vi "Main_16b_DNAtts for speed compare.vi"() -> ()   [LabVIEW 2023]
uses:
  ENUM_Direction.ctl
  07240289-bc54-4016-8294-605637801abb.vi
panel:
  out "x-y":i32
  out "answer":i32
  in  "Puzzle":string="\\.......................|..-.............../../.......|...............\\.\\.....|..../.............|............\n........................../....../..............................-............-.-..--.........-...........\\/...\n....\\............../...........-...-......|.............................\\...............-........-....|.......\n......\\....|................./.\\................/..................../.......................|..\\......-......\n.................../..................-./.................../.....-...................|......\\.......|\\...\\./.\n.....|........../....................\\../..\\.../.\\.......-.............\\...........\\......|.\\..-..........-...\n..../............/.....\\...................../..--\\........|......\\....-...|.-...../......-........../........\n..............\\.-............./........./....|\\.......\\..........|.................|.|.................-......\n.....|..........-................-.../..........-........................\\.......|.........................-..\n.|.-......./....................\\........-.............../..\\.|.-\\...........\\./.................-............\n................|/............................../..-.\\..................-..../../...../.../..../..........|...\n........................./.....................\\..\\....-....../-.....................\\|.........././.-........\n...\\.....................-...../|............--......-..|...../.....|......|.../.\\....|.............\\|.......\\\n.........-...-.....|.........../...-/........|......./|............-.......-.....\\.............\\|....../......\n.....|...|.................|...../.............|.................../..........\\|..\\......|..|....-............\n...........................-.........\\......\\.............\\...................-.....-.\\.......-.....|.........\n.................-.............-......./.............-..\\./......|....-..-..........-....-............\\.......\n.\\..\\.......-......|........................\\.............-.......................|.........|\\.|..\\......--/..\n..........-.....||--........|........-....../...........|../...-.........../.....-.\\..........|.......-.......\n..........\\..........|..................\\.................-..../............/..........|.......-........../...\n..--......../..........-..|........./.........-...../........-.................|..\\............../.....-......\n.....\\.............|...../......../............./||..........................\\............|...................\n..-.................-|..-....................\\.................|...\\.....\\............./......-.......\\.......\n............-../......\\...../.-....-.....-....-./../......\\..|..|............................|.../..|.........\n-................./................................................|...............|....|.....-.....|....../..\n...........-...................|...........\\.......-..\\.......-...........|..-....../........|...............|\n.........|...|-........../...-..........|.........\\.....||......./....|...............\\......-......\\...../...\n....|.........|............\\.-.......................................-.......................|.-..|.\\...\\.-...\n.|....|....-/....................\\\\..........................|........\\|...|..............\\..|......-.\\../....\n..|.\\......|..../.....|.......-....................|.\\..\\............/......................|.....\\../../.....\n.......|\\\\.\\/......................./.............|................../.........|.....\\-.......................\n......................................../.../................\\-..............-................./......\\.......\n............../............/\\......./........................./......|............\\/..........................\n......./................|......../.........-............\\.../.|....../....|...../..../......../...............\n...................|............-\\........../...\\.......\\....\\.....-.........-./....|.........................\n.....-..-\\.................|\\...........................|..........\\........-...|.............................\n..............................-.............-.......\\......................../.......\\|.......|...-....-......\n\\...................\\..../.................\\................|......-...-............./.-......................\n........................./.|./...|..\\.-............|.-.....-..........\\....-..../.....|.......|...............\n.................../......../..................|.|...............|.......|\\.....|......|...............\\/..|..\n.........|....-......../........-./..|.../..|./...................-........|..................................\n..|../............-......-.........................-..|....-................-..\\....../...........|...........\n....................-...............|.../.....|..../......../...|.......\\.....-.....\\..............-..\\.-.....\n...........\\.........../............................................\\......-................-.......|.....-...\n..-............./.......-\\...........|-..-../............../................................../...............\n.................\\.......\\............../.|.......-...\\............................................\\.-........\n.\\....|....\\......|........./.....--......................................|................\\..|-..............\n......../...............-..........................|...........................-.............-\\.-..|..........\n.......|......|/...\\........./......../.....\\.........\\.......................-...........\\..\\................\n.-..-../.............|................./../.................\\........-......|.\\.....||...................\\|...\n/......../....\\.....|-..........\\..............-.....|............/\\......\\...//....................\\...-/....\n................-...........-.-\\-..........\\.-./......../-................./../.\\........................./...\n-.........-.....|.....-..|..|.........|...................-..........\\/.-.....................................\n......./...../......\\............-.|...............|..../.........|....\\.................../..............|...\n...........|.......|....|...............\\........................\\/..\\......................................\\.\n......\\........-.........................\\..........\\.............\\......................\\/.....\\..|..........\n......\\...........|.........../..-............./........................../...-......../...............\\..|...\n..|............\\../........../............\\...|.......................-...............\\-../.|...|\\.....\\......\n.|....\\.|....-|.........\\......./.................../.|........|....../.--.\\.....\\..............-\\\\.........-.\n......................./.......\\...........|.\\............-.....\\.............\\.........--......../.\\..-.|../.\n......../.............../......\\.\\....|.............../...........................-........-......../.........\n.......|\\.............|.../|/........../....\\.....-....|.............-......./........\\..\\........\\..|......-.\n.............../...........-.....\\..\\....-...../...|......\\...........................\\...|...........|/......\n.............|....../.................../..|.....................|.......|....//..............\\...............\n......./....\\............................-.........................-/......../|......-....|.............../...\n...........................|...................\\...............................-.................|...........\\\n.............................-......./..../...................\\.../...........-.|......................||.....\n\\....\\....\\...-./......../.........\\................./................\\...................|...........-.......\n................-.../............/\\..................\\.\\..-....../................./..........|...............\n......../...\\.......................\\.......\\..\\......|.....|../..........\\..........-.............|..........\n../.........................................-\\..........-.........|-./.....-...|..|.......\\........-...../../.\n.....|..........-......../|-..............|.................-...........|...\\.....................\\...........\n.......|..............\\....\\.....-............../..\\\\..\\.......-........./.........-..|...|................../\n..........-.......-.-................../.........\\\\...../.....|..........\\......./.|.............-...........\\\n..................................-..................|...........\\../\\...../..../...\\................/........\n...-.........................................................\\.|..............\\..................\\............\n-.|..|...................../../.|.......\\.....|.....\\.\\...\\.........-.................................../.....\n...\\./....../........\\.......-.................\\.........|............-.........../...........\\.|.........|.\\.\n..........-...\\.............-.-............-.-................/.....................|........|............-...\n|......./............/..|..............\\...............|.......|\\................/....|.........|.........\\..\\\n.....\\../\\./.....................-.............\\..................|.|.........................................\n............/......../.../.......\\............/.........................\\........................\\............\n....../..|.............../....................-.......\\................................................|.....\\\n................................../.......././.......\\.....|.\\......-.........-..||......../........-.//......\n........................\\.......|............-....-...../..............................-............-....|...-\n.....-.......|......\\..|.........-....|......\\......../..../.......\\..........|....\\.............||..\\........\n..........|...........-|.......\\.......-....../...../..........||.......................\\............-..|.....\n.................../../..............................|....|................/........|-....|................/..\n.....................\\................/............................/-........./...|.............\\...|..|\\.....\n.....\\..\\..........\\......../......|.........-....-..-..|...........\\....|./....\\.\\..\\............../.........\n.......-...............-....../...........-.......................|../...............|...|.........../..../...\n.............|.../..................\\..\\..........-........||................\\/...........-|..................\n.............-..............-\\.../.................|......\\...../..........\\...-.....-....../................\\\n.....-....................................-.........\\/............../.............................|...........\n./.|../......\\\\..........................................|..............\\|/..-\\..........................\\....\n...........-.........\\............./....-........-....-....-.........\\..\\....-\\...-...............--.........-\n..\\.............................\\............................./\\..........-.............-...-./........../....\n.................../........\\....|..-....|||./..............-......-./....................../..|...|..........\n......\\.........../............|\\...|.-................../....................|\\..|..\\.............-./......|.\n...........-...................-.|........................\\...............|/..-...\\...|/\\...........|.........\n............|..../..................................\\.......................\\........................-........\n.\\..........................|......|......../.|....................../.......\\......\\.............../.........\n..........-.../............/..........................|....-......................|.-................|.-......\n......../............-...|.....|......../-.....-|...|./.......-..................-\\...........................\n...............\\.\\/.-....././................-.../..../.............../-|.....-.......|......./..--...........\n..........-\\\\.|-................./../..|.-.....--................../.................../.|.......-............\n..\\.................-..............-...............\\.....|......................./..\\.....--........./..../..\\\n.......-....../..............|..................\\....|..|..........-.....|.|.-.........................\\......\n..../..\\...\\....................................||.|......................................|.......\\/.........-\n................\\-.-.....||....\\.........................-...................................................|"
  in  "Example":string=".|...\\....\n|.-.\\.....\n.....|-...\n........|.\n..........\n.........\\\n..../.\\\\..\n.-.-/..|..\n.|....-|.\\\n..//.|...."
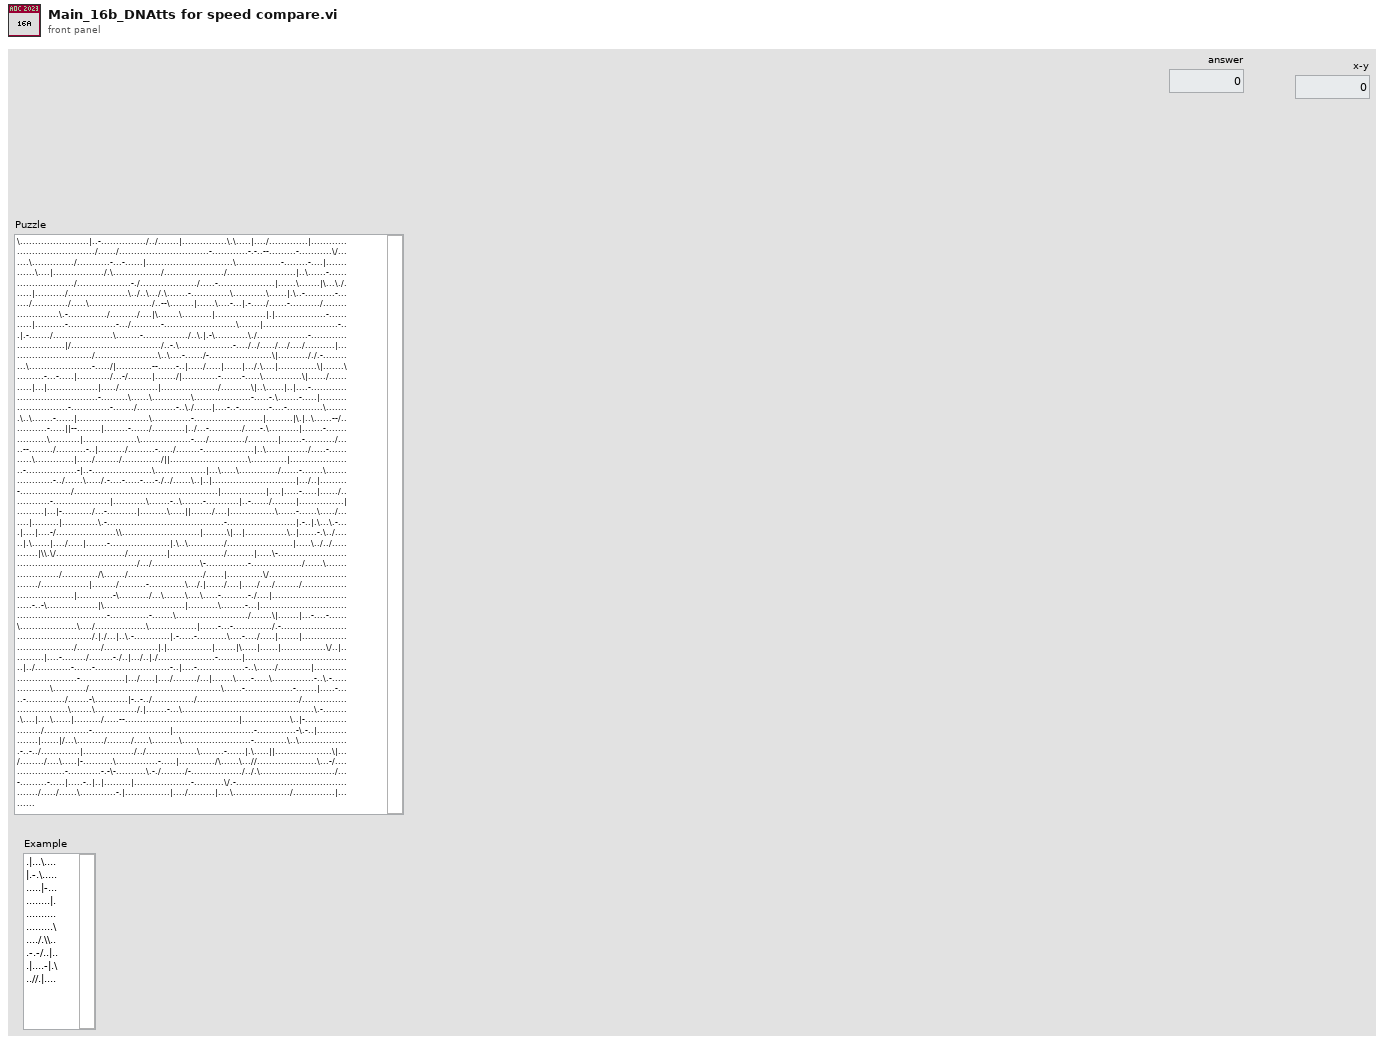
[diagram p1: front panel]
types:
  T1 = typedef "ENUM_Direction.ctl" = enum16{"Up", "Left", "Down", "Right"}
  T2 = cluster{"number of columns":i32, i32, "Direction":T1}
  T3 = cluster{"number of columns":i32, "matrix":i32, "Direction":T1}[]
  T4 = cluster{"number of columns":i32, "matrix":i32, "Direction":T1}
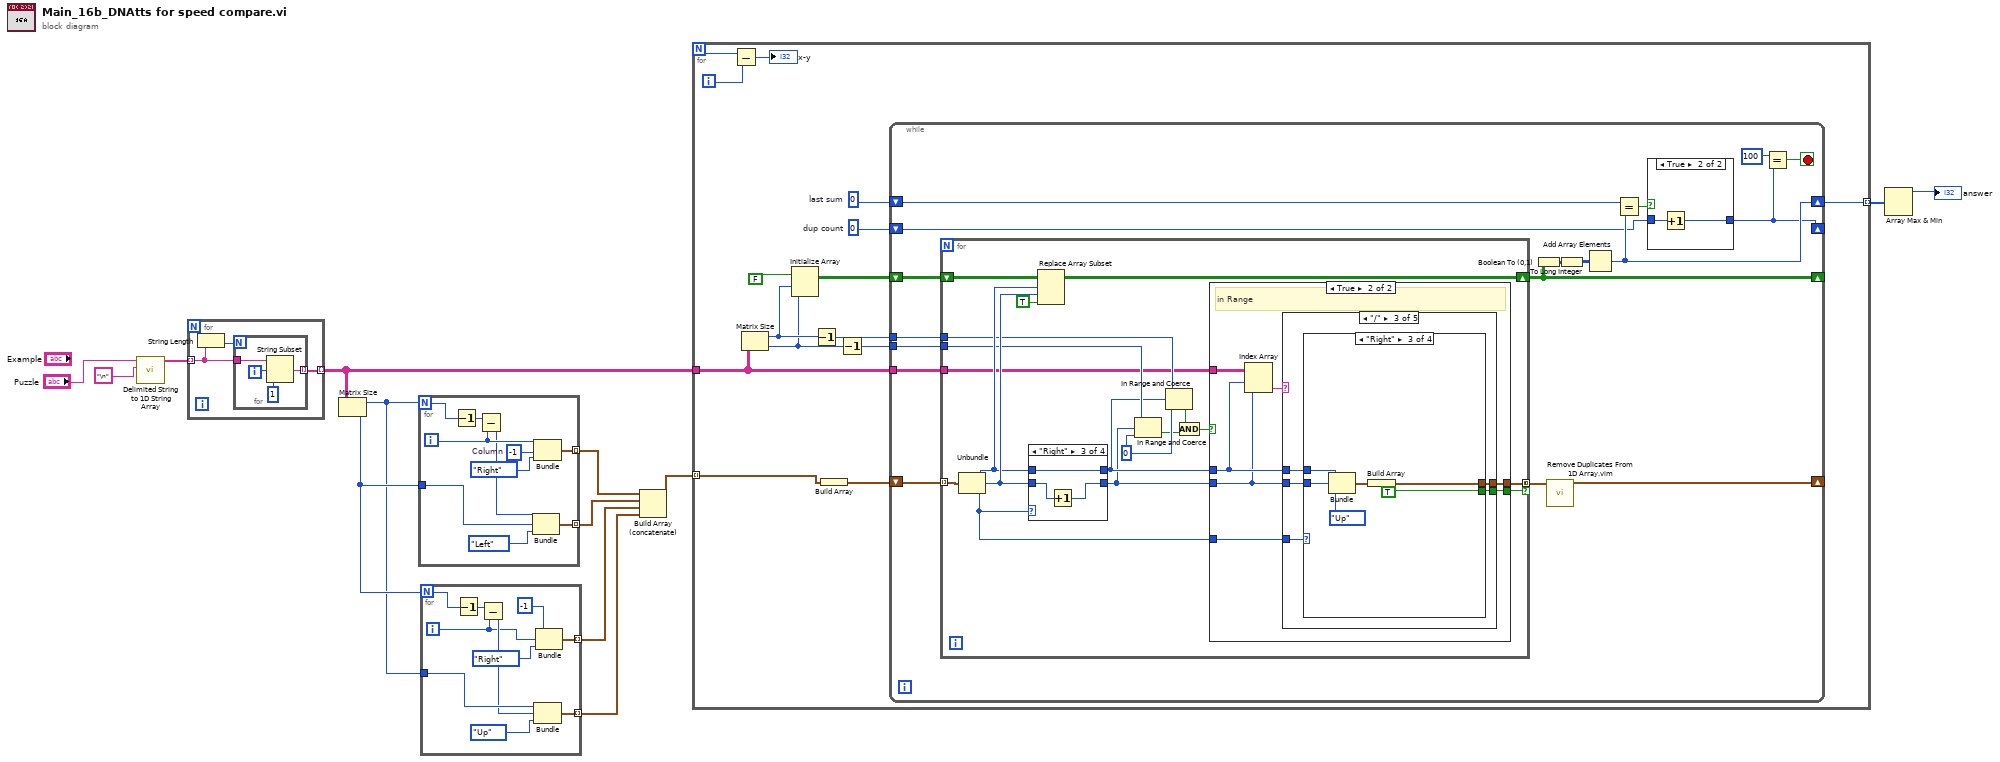
[diagram p0: block diagram]
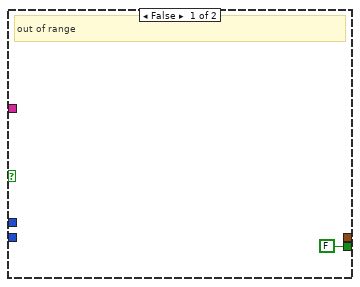
[diagram p3: hidden frame]
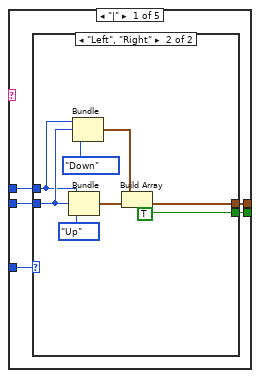
[diagram p4: hidden frame]
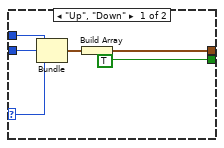
[diagram p5: hidden frame]
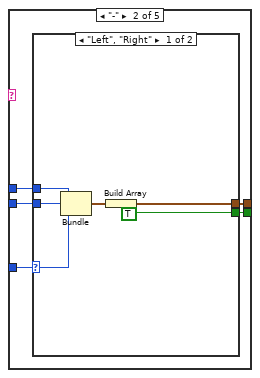
[diagram p6: hidden frame]
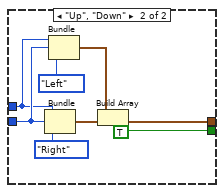
[diagram p7: hidden frame]
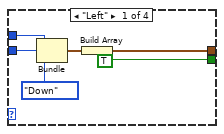
[diagram p8: hidden frame]
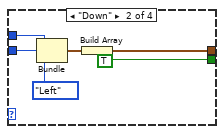
[diagram p9: hidden frame]
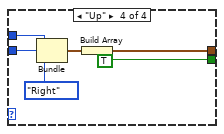
[diagram p10: hidden frame]
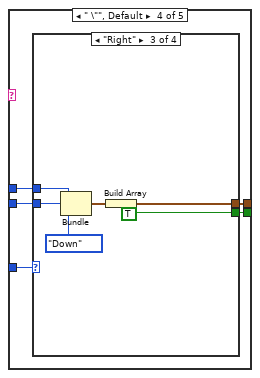
[diagram p11: hidden frame]
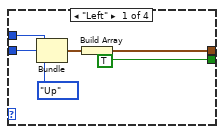
[diagram p12: hidden frame]
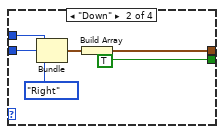
[diagram p13: hidden frame]
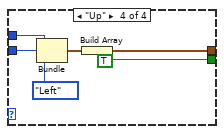
[diagram p14: hidden frame]
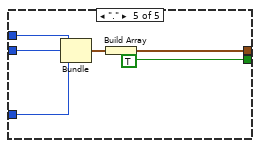
[diagram p15: hidden frame]
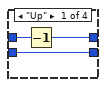
[diagram p16: hidden frame]
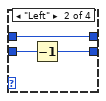
[diagram p17: hidden frame]
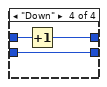
[diagram p18: hidden frame]
diagram:
  n1 = call <vilib>:"Delimited String to 1D String Array.vi"("delimiter"="\n", "delimited string"="Puzzle") -> ("string array"=w12:string[])  [unwired: 9 in]
  n2 = for {
    tunnel: w12 -> [w15] mode=indexing
    tunnel: [w14] -> w7 mode=indexing
    n3 = String Length(string=w15) -> (length=w16:i32)
    n4 = for {
      N: w16 -> [_]
      tunnel: w15 -> [w20]
      tunnel: [w17] -> w14 mode=indexing
      i -> [w19]
      n5 = String Subset(string=w20, offset (0)=w19, length (rest)=1 ("length (rest)")) -> (substring=w17:string)
    }
  }
  n6 = Matrix Size(0:w7) -> (1:w3:i32, 2:w4:i32)
  n7 = for {
    N: w3 -> [w30]
    tunnel: w4 -> [w22]
    tunnel: [w25] -> w6 mode=indexing
    tunnel: [w21] -> w5 mode=indexing
    i -> [w26]
    w28 = -1  # Column
    n8 = Decrement(x=w30) -> (x-1=w29:i32)
    n9 = Subtract(x=w29, y=w26) -> (x-y=w23:i32)
    n10 = Bundle(w23, "matrix"=w22, "Direction"=ENUM_Direction."Left") -> (w21:cluster{i32, "matrix":i32, "Direction":T1})  [unwired: 1 in]
    n11 = Bundle(w26, "Column"=w28, "Direction"=ENUM_Direction."Right") -> (w25:cluster{i32, "Column":i32, "Direction":T1})  [unwired: 1 in]
  }
  n12 = for {
    N: w4 -> [w40]
    tunnel: w3 -> [w34]
    tunnel: [w37] -> w2 mode=indexing
    tunnel: [w35] -> w1 mode=indexing
    i -> [w32]
    n13 = Decrement(x=w40) -> (x-1=w39:i32)
    n14 = Subtract(x=w39, y=w32) -> (x-y=w33:i32)
    n15 = Bundle("number of columns"=w34, w33, "Direction"=ENUM_Direction."Up") -> (w35:T2)  [unwired: 1 in]
    n16 = Bundle(-1, w32, "Direction"=ENUM_Direction."Right") -> (w37:cluster{i32, i32, "Direction":T1})  [unwired: 1 in]
  }
  n17 = Build Array (concatenate)(w6, w5, w2, w1) -> (w8:T3)
  n18 = for {
    N -> [w43]
    tunnel: w7 -> [w47]
    tunnel: [w45] -> w10 mode=indexing
    tunnel: w8 -> [w44] mode=indexing
    i -> [w42]
    w51 = 0  # dup count
    w52 = 0  # last sum
    n19 = Subtract(x=w43, y=w42) -> (x-y=→"x-y":i32)
    n20 = Matrix Size(0:w47) -> (1:w54:i32, 2:w53:i32)
    n21 = Initialize Array(FALSE, w54, w53) -> (w50:bool[][])
    n22 = Decrement(x=w54) -> (x-1=w49:i32)
    n23 = Build Array(w44) -> (w46:T3)
    n24 = Decrement(x=w53) -> (x-1=w48:i32)
    n25 = while {
      shift-right: [w62] -> w45
      shift-left: w52 -> [w61]
      shift-right: [w58] -> _
      shift-left: w51 -> [w59]
      shift-right: [w65] -> _
      shift-left: w50 -> [w72]
      tunnel: w49 -> [w70]
      tunnel: w48 -> [w69]
      tunnel: w47 -> [w68]
      shift-right: [w66] -> _
      shift-left: w46 -> [w71]
      stop <- w56 stop-if-true
      n26 = for {
        shift-right: [w92] -> w65
        shift-left: w72 -> [w93]
        tunnel: w71 -> [w91] mode=indexing
        tunnel: w70 -> [w87]
        tunnel: w69 -> [w86]
        tunnel: w68 -> [w81]
        tunnel: [w77] -> w67 mode=concatenating if=w76
        w85 = 0 ("lower limit")
        n27 = Unbundle(w91) -> ("number of columns"=w88:i32, "matrix"=w89:i32, "Direction"=w78:T1)
        n28 = case shown="\"Right\"" w78 {
          tunnel: w89 -> [w205 w209 w212 w214]
          tunnel: w88 -> [w206 w208 w211 w215]
          tunnel: [w205 w207 w210 w214] -> w79
          tunnel: [w204 w208 w211 w213] -> w80
          frame "Up" {
            n29 = Decrement(x=w206) -> (x-1=w204:i32)
          }
          frame "Left" {
            n30 = Decrement(x=w209) -> (x-1=w207:i32)
          }
          frame "Right" {
            n31 = Increment(x=w212) -> (x+1=w210:i32)
          }
          frame "Down" {
            n32 = Increment(x=w215) -> (x+1=w213:i32)
          }
        }
        n33 = Replace Array Subset(array=w93, new element=TRUE ("new element/subarray"), index (row)=w88, index (col)=w89) -> (w92:bool[][])
        n34 = In Range and Coerce(upper limit=w86, x=w79, lower limit=w85) -> (In Range?=w83:bool)  [unwired: 1 out]
        n35 = In Range and Coerce(upper limit=w87, x=w80, lower limit=w85) -> (In Range?=w84:bool)  [unwired: 1 out]
        n36 = And(x=w84, y=w83) -> (x .and. y?=w82:bool)
        n37 = case shown="True" w82 {
          tunnel: w81 -> [_ w101]
          tunnel: w80 -> [_ w98]
          tunnel: w79 -> [_ w97]
          tunnel: w78 -> [_ w99]
          tunnel: [_ w96] -> w77
          tunnel: [FALSE w95] -> w76
          frame False {
            # "out of range"
          }
          frame True {
            # "in Range"
            n38 = Index Array(array=w101, index (row)=w98, index (col)=w97) -> (element=w100:string)
            n39 = case shown="\"/\"" w100 {
              tunnel: w99 -> [w106 w125 w144 w173 w203]
              tunnel: w98 -> [w105 w124 w143 w172 w202]
              tunnel: w97 -> [w104 w123 w142 w171 w201]
              tunnel: [w103 w122 w141 w170 w200] -> w96
              tunnel: [w102 w121 w140 w169 TRUE] -> w95
              frame "|" {
                n40 = case shown="\"Left\", \"Right\"" w106 {
                  selector: w106 -> [w110 _]
                  tunnel: w105 -> [w111 w114]
                  tunnel: w104 -> [w112 w115]
                  tunnel: [w108 w119] -> w103
                  tunnel: [TRUE TRUE] -> w102
                  frame "Up", "Down" {
                    n41 = Bundle("number of columns"=w111, "matrix"=w112, "Direction"=w110) -> (w109:T4)  [unwired: 1 in]
                    n42 = Build Array(w109) -> (w108:T3)
                  }
                  frame "Left", "Right" {
                    n43 = Bundle("number of columns"=w114, "matrix"=w115, "Direction"=ENUM_Direction."Up") -> (w120:T4)  [unwired: 1 in]
                    n44 = Bundle("number of columns"=w114, "matrix"=w115, "Direction"=ENUM_Direction."Down") -> (w113:T4)  [unwired: 1 in]
                    n45 = Build Array(w113, w120) -> (w119:T3)
                  }
                }
              }
              frame "-" {
                n46 = case shown="\"Left\", \"Right\"" w125 {
                  selector: w125 -> [w129 _]
                  tunnel: w124 -> [w130 w133]
                  tunnel: w123 -> [w131 w134]
                  tunnel: [w127 w138] -> w122
                  tunnel: [TRUE TRUE] -> w121
                  frame "Left", "Right" {
                    n47 = Bundle("number of columns"=w130, "matrix"=w131, "Direction"=w129) -> (w128:T4)  [unwired: 1 in]
                    n48 = Build Array(w128) -> (w127:T3)
                  }
                  frame "Up", "Down" {
                    n49 = Bundle("number of columns"=w133, "matrix"=w134, "Direction"=ENUM_Direction."Right") -> (w139:T4)  [unwired: 1 in]
                    n50 = Bundle("number of columns"=w133, "matrix"=w134, "Direction"=ENUM_Direction."Left") -> (w132:T4)  [unwired: 1 in]
                    n51 = Build Array(w132, w139) -> (w138:T3)
                  }
                }
              }
              frame "/" {
                n52 = case shown="\"Right\"" w144 {
                  tunnel: w143 -> [w149 w155 w161 w167]
                  tunnel: w142 -> [w150 w156 w162 w168]
                  tunnel: [w147 w153 w159 w165] -> w141
                  tunnel: [TRUE TRUE TRUE TRUE] -> w140
                  frame "Left" {
                    n53 = Bundle("number of columns"=w149, "matrix"=w150, "Direction"=ENUM_Direction."Down") -> (w148:T4)  [unwired: 1 in]
                    n54 = Build Array(w148) -> (w147:T3)
                  }
                  frame "Down" {
                    n55 = Bundle("number of columns"=w155, "matrix"=w156, "Direction"=ENUM_Direction."Left") -> (w154:T4)  [unwired: 1 in]
                    n56 = Build Array(w154) -> (w153:T3)
                  }
                  frame "Right" {
                    n57 = Bundle("number of columns"=w161, "matrix"=w162, "Direction"=ENUM_Direction."Up") -> (w160:T4)  [unwired: 1 in]
                    n58 = Build Array(w160) -> (w159:T3)
                  }
                  frame "Up" {
                    n59 = Bundle("number of columns"=w167, "matrix"=w168, "Direction"=ENUM_Direction."Right") -> (w166:T4)  [unwired: 1 in]
                    n60 = Build Array(w166) -> (w165:T3)
                  }
                }
              }
              frame " \"", Default {
                n61 = case shown="\"Right\"" w173 {
                  tunnel: w172 -> [w178 w184 w190 w196]
                  tunnel: w171 -> [w179 w185 w191 w197]
                  tunnel: [w176 w182 w188 w194] -> w170
                  tunnel: [TRUE TRUE TRUE TRUE] -> w169
                  frame "Left" {
                    n62 = Bundle("number of columns"=w178, "matrix"=w179, "Direction"=ENUM_Direction."Up") -> (w177:T4)  [unwired: 1 in]
                    n63 = Build Array(w177) -> (w176:T3)
                  }
                  frame "Down" {
                    n64 = Bundle("number of columns"=w184, "matrix"=w185, "Direction"=ENUM_Direction."Right") -> (w183:T4)  [unwired: 1 in]
                    n65 = Build Array(w183) -> (w182:T3)
                  }
                  frame "Right" {
                    n66 = Bundle("number of columns"=w190, "matrix"=w191, "Direction"=ENUM_Direction."Down") -> (w189:T4)  [unwired: 1 in]
                    n67 = Build Array(w189) -> (w188:T3)
                  }
                  frame "Up" {
                    n68 = Bundle("number of columns"=w196, "matrix"=w197, "Direction"=ENUM_Direction."Left") -> (w195:T4)  [unwired: 1 in]
                    n69 = Build Array(w195) -> (w194:T3)
                  }
                }
              }
              frame "." {
                n70 = Bundle("number of columns"=w202, "matrix"=w201, "Direction"=w203) -> (w198:T4)  [unwired: 1 in]
                n71 = Build Array(w198) -> (w200:T3)
              }
            }
          }
        }
      }
      n72 = Boolean To (0,1)(Boolean=w65) -> (0, 1=w64:i16[][])
      n73 = call "Remove Duplicates From 1D Array.vim"("array"=w67) -> ("array with duplicates removed"=w66:T3)  [unwired: 10 in]
      n74 = To Long Integer(number=w64) -> (32bit integer=w63:i32[][])
      n75 = Add Array Elements(numeric array=w63) -> (sum=w62:i32)
      n76 = Equal?(x=w61, y=w62) -> (x = y?=w60:bool)
      n77 = case shown="True" w60 {
        tunnel: w59 -> [w73 w75]
        tunnel: [w73 w74] -> w58
        frame False {
        }
        frame True {
          n78 = Increment(x=w75) -> (x+1=w74:i32)
        }
      }
      n79 = Equal?(x=100, y=w58) -> (x = y?=w56:bool)
    }
  }
  n80 = Array Max & Min(array=w10) -> (max value=→"answer":i32)  [unwired: 3 out]
